vi "Write Friction Coefficient.vi"(8 "error in":errorcluster, 10 "Friction Coefficient":dbl, 11 "Friction in":refnum<class "Friction.lvclass">) -> (0 "error out":errorcluster, 3 "Friction out":refnum<class "Friction.lvclass">)   [LabVIEW 2016, in "Friction.lvclass"]
uses:
  Friction.lvclass
  Friction.lvclass/Friction.ctl
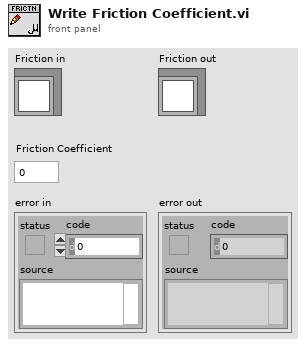
[diagram p1: front panel]
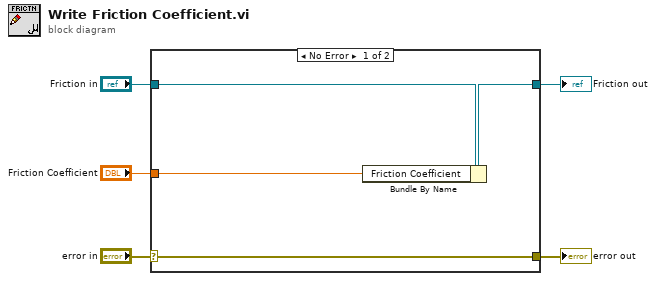
[diagram p0: block diagram]
diagram:
  n1 = case shown="No Error" "error in" {
    selector: "error in" -> [w9 w10]
    tunnel: [w9 w10] -> w4
    tunnel: [w7 w11] -> w2
    tunnel: "Friction in" -> [w8 w11]
    tunnel: "Friction Coefficient" -> [w6 _]
    frame No Error {
      n2 = Bundle By Name(cluster=w8, "Friction Coefficient"=w6) -> (w7:refnum<class "Friction.lvclass">)
    }
    frame Error {
    }
  }
  "error out" <- w4
  "Friction out" <- w2
